vi "Main.vi"(0 "Set busy":bool, 5 "icon":u16(ring), 11 "Error in":errorcluster) -> (15 "Error out":errorcluster)   [LabVIEW 2020, in "Cursor.lvlib"]
doc: "This VI is basically used as implementation of cursors of setting the cursor busy for a specified time."
uses:
  Cursor.lvlib
  <vilib>/Utility/cursorutil.llb/Set Cursor (Icon Pict).vi
panel:
  # "SET BUSY"
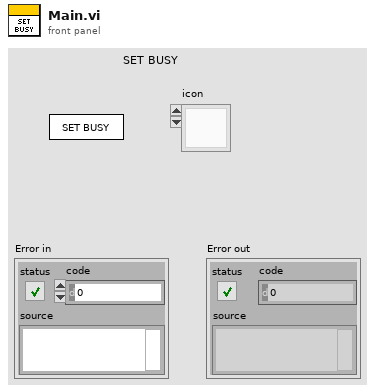
[diagram p1: front panel]
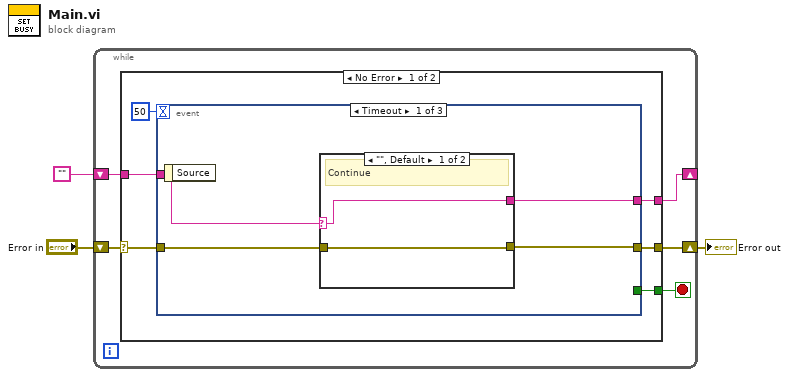
[diagram p0: block diagram]
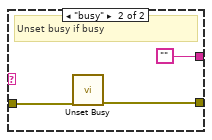
[diagram p2: hidden frame]
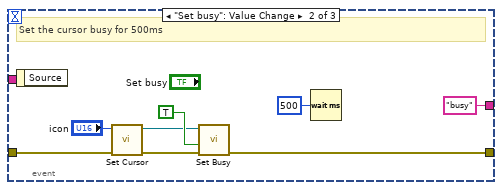
[diagram p3: hidden frame]
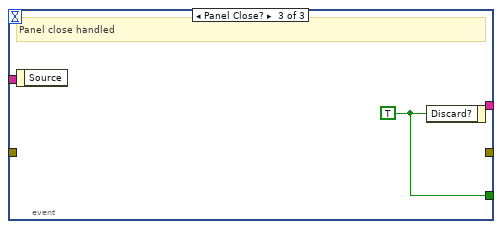
[diagram p4: hidden frame]
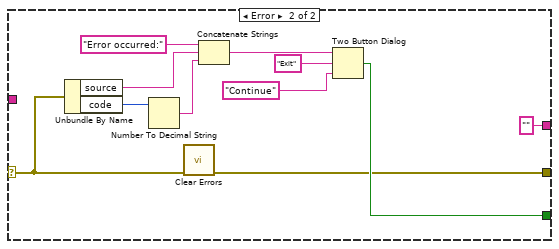
[diagram p5: hidden frame]
diagram:
  n1 = while {
    shift-right: [w7] -> w2
    shift-left: "Error in" -> [w8]
    shift-right: [w4] -> _
    shift-left: "" -> [w5]
    stop <- w6 stop-if-true
    n2 = case shown="No Error" w8 {
      selector: w8 -> [w14 w43]
      tunnel: [w13 w34] -> w7
      tunnel: [w12 w35] -> w6
      tunnel: w5 -> [w10 _]
      tunnel: [w9 ""] -> w4
      frame No Error {
        n3 = event shown="[0] Timeout" {
          selector: _ -> [_ _ _]
          dyn-events: _ -> [_ _ _]
          timeout: 50 -> [_ _ _]
          tunnel: [w15 w29 _] -> w13
          tunnel: w14 -> [w18 w27 _]
          tunnel: [_ _ w32] -> w12
          tunnel: w10 -> [w17 _ _]
          tunnel: [w16 "busy" _] -> w9
          event Timeout {
            n4 = event-data() -> ()  [unwired: 1 in, 1 out]
            n5 = case shown="\"\", Default" w17 {
              selector: w17 -> [w20 _]
              tunnel: w18 -> [w19 w22]
              tunnel: [w20 ""] -> w16
              tunnel: [w19 w21] -> w15
              frame "", Default {
                # "Continue"
              }
              frame "busy" {
                # "Unset busy if busy"
                n6 = call <vilib>:"Unset Busy.vi"("error in (no error)"=w22) -> ("error out"=w21:errorcluster)  [unwired: 10 in]
              }
            }
          }
          event "Set busy": Value Change {
            # "Set the cursor busy for 500ms"
            n7 = event-data() -> ()  [unwired: 1 in, 1 out]
            n8 = call-poly <vilib>:"Set Cursor.vi"("error in (no error)"=w27, "icon"="icon") -> ("error out"=w26:errorcluster, "previous cursor ID"=w24:refnum<k1>)  [unwired: 8 in]
            n9 = call <vilib>:"Set Busy.vi"("error in (no error)"=w26, "disable click? (T)"=TRUE, "cursor ID"=w24) -> ("error out"=w29:errorcluster)  [unwired: 7 in, 1 out]
            n10 = Wait (ms)(milliseconds to wait=u32 500) -> ()  [unwired: 1 out]
          }
          event Panel Close? {
            w32 = TRUE ("Discard?")
            # "Panel close handled"
            n11 = event-data() -> ()  [unwired: 1 in, 1 out]
            n12 = event-data("Discard?"=w32) -> ()  [unwired: 1 in, 1 out]
          }
        }
      }
      frame Error {
        n13 = Unbundle By Name(w43) -> ("source"=w41:string, "code"=w40:i32)
        n14 = Number To Decimal String(number=w40) -> (decimal integer string=w39:string)  [unwired: 1 in]
        n15 = call <vilib>:"Clear Errors.vi"("error in (no error)"=w43) -> ("error out"=w34:errorcluster)  [unwired: 5 in, 1 out]
        n16 = Concatenate Strings("Error occurred:" ("string"), w41, w39) -> (w38:string)
        n17 = Two Button Dialog(message=w38, 1:"Continue" ("F button name (\"Cancel\")"), 2:"Exit" ("T button name (\"OK\")")) -> (T button?=w35:bool)
      }
    }
  }
  "Error out" <- w2
